vi "bosch 4-9 Nernst T to R.vi"(10 "T":dbl) -> (2 "R":dbl)   [LabVIEW 2014, in "UEGO Sim Engine.lvlib"]
uses:
  UEGO Sim Engine.lvlib
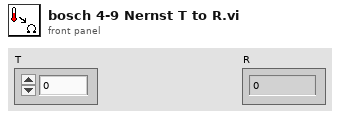
[diagram p1: front panel]
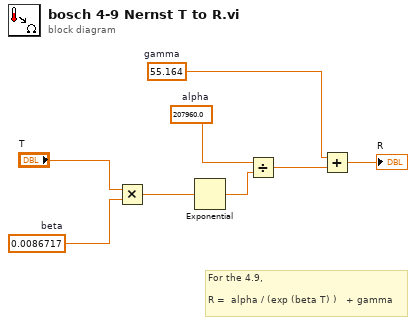
[diagram p0: block diagram]
diagram:
  w7 = 0.0086717  # beta
  w5 = 207960.0  # alpha
  w2 = 55.164  # gamma
  # "For the 4.9, \n\nR =  alpha / (exp (beta T) )   + gamma"
  n1 = Multiply(x="T", y=w7) -> (x*y=w6:dbl)
  n2 = Exponential(1:w6) -> (0:w4:dbl)
  n3 = Divide(x=w5, y=w4) -> (x/y=w3:dbl)
  n4 = Add(x=w2, y=w3) -> (x+y=→"R":dbl)
